vi "rs3 get error message.vi"(8 "error in (no error)":errorcluster, 11 "error in":u64) -> (0 "error out":errorcluster, 2 "error out":u64, 3 "error message":string)   [LabVIEW 2023]
doc: "const char * rs_get_error_message (const rs_error * error);"
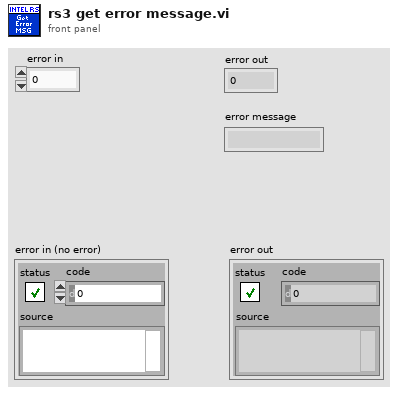
[diagram p1: front panel]
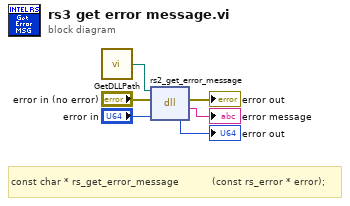
[diagram p0: block diagram]
diagram:
  # "const char * rs_get_error_message           (const rs_error * error);"
  n1 = call "GetDLLPath.vi"() -> ("DLL Path"=w1:path)
  n2 = dll-call lib="C:/STEAMSyndicate/RealSenseWrappers/VI Wrappers (add ons) Public/RealSense/realsense2.dll" fn="rs2_get_error_message"(path in=w1, error in="error in (no error)", "error"="error in") -> (error out=→"error out":errorcluster, "return type"=→"error message":string, "error"=→"error out":u64)  [unwired: 1 in, 1 out]
